vi "Test - Is VeriStand Running.vi"() -> ()   [LabVIEW 2015]
uses:
  <vilib>/NI Veristand/Execution/Workspace/NI_VS Workspace ExecutionAPI.lvlib
panel:
  out "error out":errorcluster
  in  "stop":bool
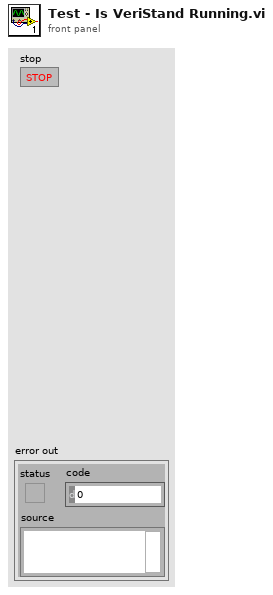
[diagram p1: front panel]
types:
  T1 = typedef "NI_VS Workspace ExecutionAPI.lvlib/WorkspaceAPI.ctl" = refnum<k24>
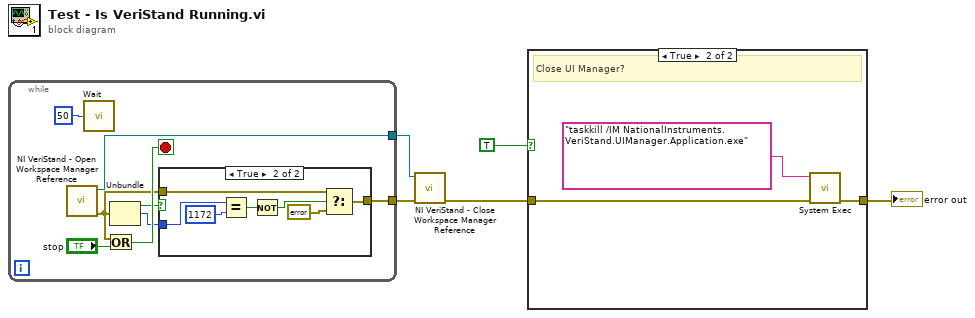
[diagram p0: block diagram]
diagram:
  n1 = while {
    tunnel: [w13] -> w5
    tunnel: [w6] -> w4
    stop <- w11 stop-if-true
    n2 = call <vilib>:"NI VeriStand - Open Workspace Manager Reference.vi"() -> ("error out"=w7:errorcluster, "WorkspaceManager"=w13:T1)  [unwired: 10 in]
    n3 = call "Wait"("Count(mSec)"=u32 50) -> ()  [unwired: 1 out]
    n4 = Or(x=w7, y="stop") -> (x .or. y?=w11:bool)
    n5 = Unbundle(w7) -> ("status"=w9:bool, "code"=w8:i32)  [unwired: 1 out]
    n6 = case shown="True" w9 {
      tunnel: w8 -> [_ w21]
      tunnel: w7 -> [w14 w16]
      tunnel: [w14 w15] -> w6
      frame False {
      }
      frame True {
        n7 = Equal?(x=w21, y=1172) -> (x = y?=w19:bool)
        n8 = Not(x=w19) -> (.not. x?=w18:bool)
        n9 = Select(t=w16, s=w18, f=errorcluster {"status"=FALSE, "code"=0, "source"=""} ("error in (no error)")) -> (s? t:f=w15:errorcluster)
      }
    }
  }
  n10 = call <vilib>:"NI VeriStand - Close Workspace Manager Reference.vi"("error in (no error)"=w4, "WorkspaceManager"=w5) -> ("error out"=w2:errorcluster)  [unwired: 9 in]
  n11 = case shown="True" TRUE {
    tunnel: w2 -> [w22 w25]
    tunnel: [w22 w24] -> w3
    frame False {
    }
    frame True {
      # "Close UI Manager?"
      n12 = call <vilib>:"System Exec.vi"("error in (no error)"=w25, "command line"="taskkill /IM NationalInstruments.VeriStand.UIManager.Application.exe" ("standard input")) -> ("error out"=w24:errorcluster)  [unwired: 6 in, 3 out]
    }
  }
  "error out" <- w3
